vi "첫TDMS코딩__쓰기.vi"   [LabVIEW 2020]
uses:
  <vilib>/Utility/sysdir.llb/System Directory Type.ctl
types:
  T1 = enum16{"open", "open or create", "create or replace", "create", "open (read-only)"}
  T2 = typedef "System Directory Type.ctl" = i32
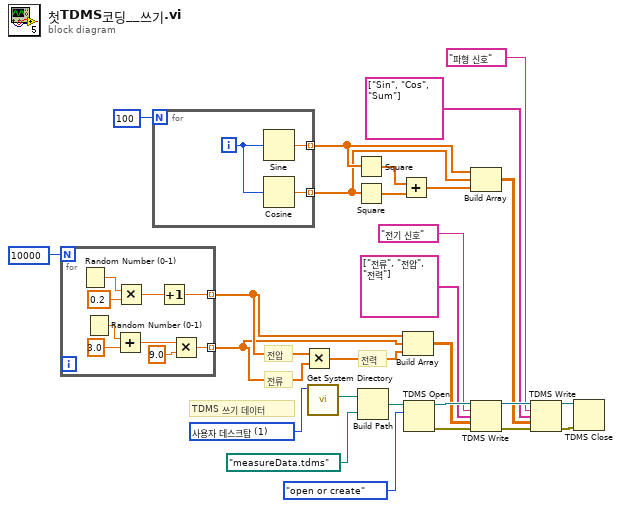
[diagram p0: block diagram]
diagram:
  w27 = T2 1 items=["사용자 홈"=0, "사용자 데스크탑"=1, "사용자 문서"=2, "사용자 어플리케이션 데이터"=3, "사용자 환경"=4, "사용자 임시"=5, "퍼블릭 문서"=6, "퍼블릭 어플리케이션 데이터"=7, "퍼블릭 환경"=8, "퍼블릭 캐시"=13, "시스템 코어 라이브러리"=9, "시스템 설치된 라이브러리"=10, "어플리케이션 파일"=11, "부팅 볼륨 루트"=12] ("system directory type")
  # "TDMS 쓰기 데이터"
  # "전력"
  # "전압"
  # "전류"
  n1 = for {
    N: 10000 -> [_]
    tunnel: [w33] -> w14 mode=indexing
    tunnel: [w28] -> w13 mode=indexing
    n2 = Random Number (0-1)() -> (number: 0 to 1=w36:dbl)
    n3 = Random Number (0-1)() -> (number: 0 to 1=w31:dbl)
    n4 = Add(x=w31, y=3.0) -> (x+y=w29:dbl)
    n5 = Multiply(x=w36, y=0.2) -> (x*y=w34:dbl)
    n6 = Increment(x=w34) -> (x+1=w33:dbl)
    n7 = Multiply(x=w29, y=9.0) -> (x*y=w28:dbl)
  }
  n8 = for {
    N: 100 -> [_]
    tunnel: [w38] -> w5 mode=indexing
    tunnel: [w37] -> w4 mode=indexing
    i -> [w39]
    n9 = Sine(x=w39) -> (sin(x)=w38:dbl)
    n10 = Cosine(x=w39) -> (cos(x)=w37:dbl)
  }
  n11 = Multiply(x=w14, y=w13) -> (x*y=w15:dbl[])
  n12 = call <vilib>:"Get System Directory.vi"("system directory type"=w27) -> ("system directory"=w26:path)  [unwired: 10 in]
  n13 = Square(x=w5) -> (x^2=w7:dbl[])
  n14 = Square(x=w4) -> (x^2=w8:dbl[])
  n15 = Build Path(base path=w26, name or relative path=path "measureData.tdms" ("이름 또는 상대 경로")) -> (appended path=w24:path)
  n16 = Add(x=w7, y=w8) -> (x+y=w6:dbl[])
  n17 = Build Array(w14, w13, w15) -> (w11:dbl[][])
  n18 = TDMS Open(10:T1."open or create" ("동작(0:open)"), 11:w24) -> (0:w22:errorcluster, 3:w23:refnum<k34>)  [unwired: 5 in]
  n19 = Build Array(w5, w4, w6) -> (w3:dbl[][])
  n20 = TDMS Write(0:w23, 5:"전기 신호", 7:string[] ["전류", "전압", "전력"], 9:w11, 11:w22) -> (4:w21:refnum<k34>, 15:w20:errorcluster)  [unwired: 1 in, 2 out]
  n21 = TDMS Write(0:w21, 5:"파형 신호", 7:string[] ["Sin", "Cos", "Sum"], 9:w3, 11:w20) -> (4:w19:refnum<k34>, 15:w18:errorcluster)  [unwired: 1 in, 2 out]
  n22 = TDMS Close(8:w18, 11:w19) -> ()  [unwired: 2 out]
